vi "Perform Double-Click Action.vi"(6 "Action":T1, 10 "Coords":T2, 11 "Debugger":refnum<class "Debugger.lvclass">) -> (0 "error out":errorcluster, 3 "Selected Actor":refnum<vi>)   [LabVIEW 2015, in "Debugger.lvclass"]
uses:
  Debugger.lvclass
  <vilib>/Utility/miscctls.llb/LVPoint32TypeDef.ctl
  Action.ctl
  Debug Tools/Actor Ref Cache/Actor Ref Cache Action.ctl
  Debugger.lvclass/Debugger.ctl
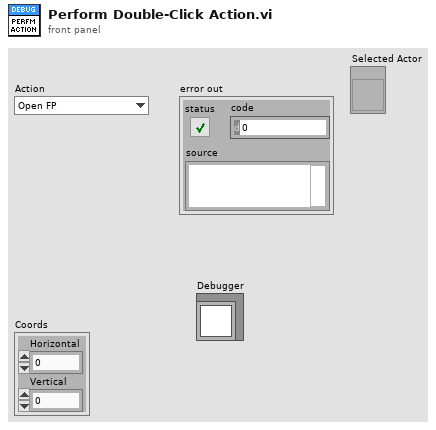
[diagram p1: front panel]
types:
  T1 = typedef "Debugger.lvclass/Action.ctl" = enum16{"Open FP", "Close FP", "Open BD", "Close BD", "Abort", "Enable Toolbar", "Move FP Up", "Move FP Down", "Move FP Left", "Move FP Right"}
  T2 = typedef "LVPoint32TypeDef.ctl" = cluster{"Horizontal":i32, "Vertical":i32}
  T3 = typedef "Actor Ref Cache Action.ctl" = enum16{"Clear", "Add Ref", "Remove Ref", "Get All Refs"}
  T4 = typedef "LVRowAndColumnTypeDef.ctl" = cluster{"Row":i32, "Column":i32}
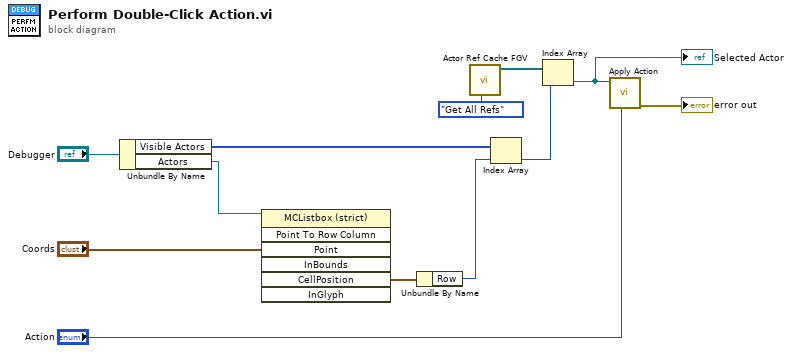
[diagram p0: block diagram]
diagram:
  n1 = Unbundle By Name("Debugger") -> ("Visible Actors"=w2:i32[], "Actors"=w1:refnum<vi>)
  n2 = invoke class="MCListbox (strict)" method="Point To Row Column"(reference=w1, "Point"="Coords") -> ("CellPosition"=w4:T4)  [unwired: 5 in, 6 out]
  n3 = Unbundle By Name(w4) -> ("Row"=w3:i32)
  n4 = call "Actor Ref Cache FGV.vi"("Action"=Actor_Ref_Cache_Action."Get All Refs") -> ("All Refs Out"=w7:refnum<vi>[])  [unwired: 10 in]
  n5 = Index Array(array=w2, index=w3) -> (element=w5:i32)
  n6 = Index Array(array=w7, index=w5) -> (element=w6:refnum<vi>)
  "Selected Actor" <- w6
  n7 = call "Apply Action.vi"("Action"="Action", "VI Refnum"=w6) -> ("error out"=→"error out":errorcluster)  [unwired: 9 in]
